vi "TeleopDriveFrwdsub.vi"(8 "SCALE":dbl=0.5 format="%#_13g", 9 "B VALUE":dbl=0.15 format="%#_13g", 10 "Deadband X value":dbl, 11 "Drive":dbl) -> (1 "Deadband FWD":bool=TRUE, 3 "Drive Output":dbl)   [LabVIEW 2017]
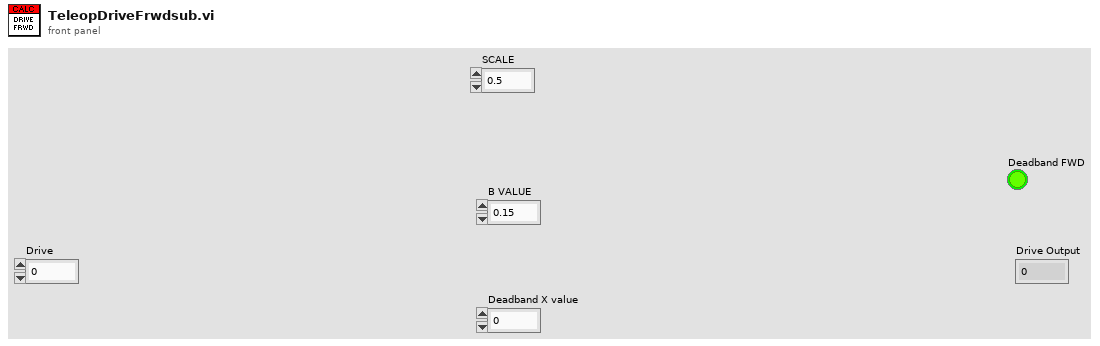
[diagram p1: front panel]
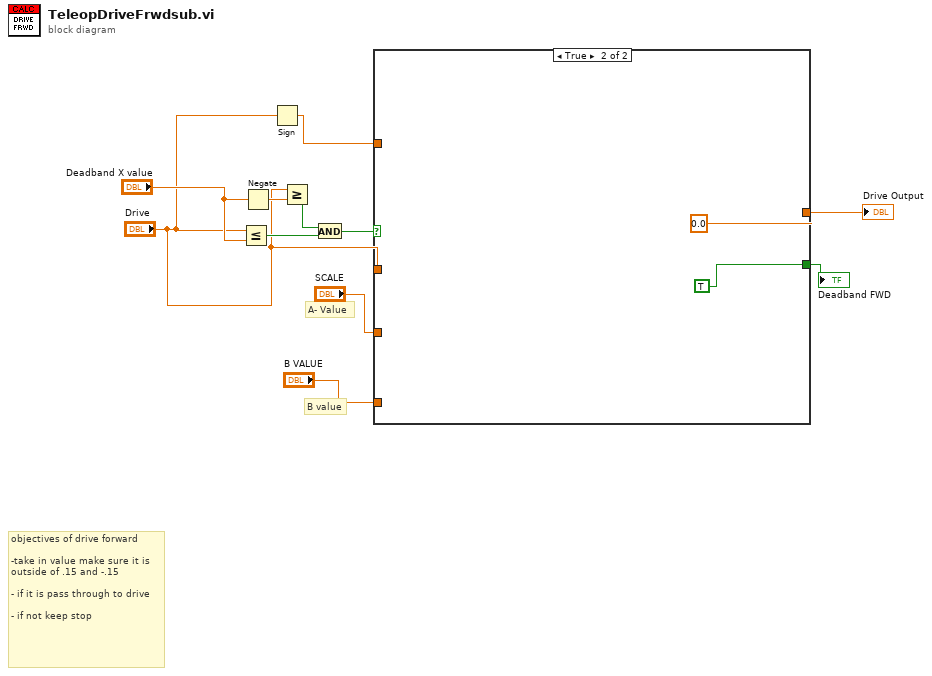
[diagram p0: block diagram]
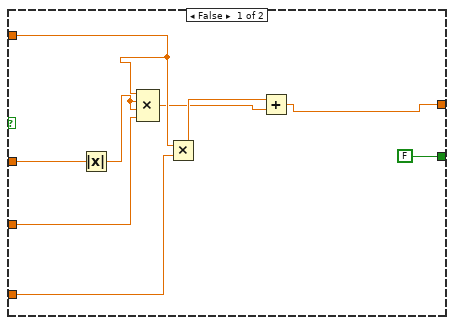
[diagram p2: hidden frame]
diagram:
  # "B value"
  # "A- Value"
  # "objectives of drive forward\n\n-take in value make sure it is \noutside of .15 and -.15\n\n- if it is pass through to drive\n\n- if not keep stop"
  n1 = Less Or Equal?(x="Drive", y="Deadband X value") -> (x <= y?=w9:bool)
  n2 = Negate(x="Deadband X value") -> (-x=w11:dbl)
  n3 = Sign(1:"Drive") -> (0:w3:dbl)
  n4 = Greater Or Equal?(x="Drive", y=w11) -> (x >= y?=w8:bool)
  n5 = And(x=w8, y=w9) -> (x .and. y?=w7:bool)
  n6 = case shown="True" w7 {
    tunnel: "Drive" -> [w13 _]
    tunnel: [w12 0.0 ("Y axis value")] -> w6
    tunnel: "SCALE" -> [w20 _]
    tunnel: "B VALUE" -> [w19 _]
    tunnel: w3 -> [w17 _]
    tunnel: [FALSE TRUE] -> w1
    frame False {
      n7 = Absolute Value(x=w13) -> (abs(x)=w14:dbl)
      n8 = Compound Arithmetic op=MULTIPLY(w17, w14, w14, w20) -> (w15:dbl)
      n9 = Multiply(x=w17, y=w19) -> (x*y=w16:dbl)
      n10 = Add(x=w16, y=w15) -> (x+y=w12:dbl)
    }
    frame True {
    }
  }
  "Drive Output" <- w6
  "Deadband FWD" <- w1
